vi "Periodic Tasks.vi"(8 "error in":errorcluster) -> ()   [LabVIEW 2013]
doc: "This VI runs in parallel to other tasks. It can contain as many user-defined periodic loops as you need. These can carry out PID or other sorts of timed response."
uses:
  <vilib>/Rock Robotics/WPI/Relay/WPI_RelayValue.ctl
  <vilib>/Rock Robotics/WPI/Solenoid/WPI_SolenoidValue.ctl
  <vilib>/Rock Robotics/WPI/Solenoid/WPI_SolenoidSetEnum.vi
  <vilib>/Rock Robotics/WPI/Solenoid/WPI_SolenoidGet.vi
  <vilib>/Rock Robotics/WPI/Solenoid/WPI_SolenoidGetEnum.vi
  <vilib>/Rock Robotics/WPI/Solenoid/Deprecated/WPI_SolenoidGetBool.vi
  <vilib>/Rock Robotics/WPI/RobotDrive/WPI_RobotDriveGetSetRefNum.vi
  Sample and Hold.vi
  <vilib>/addons/control/pid/pid.llb/PID (DBL).vi
  Stable.vi
  <vilib>/Rock Robotics/WPI/RobotDrive/WPI_RobotDriveMecanumDrive_Cartesian.vi
  <vilib>/Rock Robotics/SystemInterfaces/Utilities/FPGA_UtilitiesLED Source.ctl
  <vilib>/Rock Robotics/SystemInterfaces/Utilities/FPGA_UtilitiesLED State.ctl
  Robot Global Data.vi
  <vilib>/addons/control/pid/NI_PID_pid.lvlib
panel:
  in  "Eval Period (sec)":dbl(knob)=0.1607904282898374 scale=0.0..1.0
  in  "Tab Control 2":T1(tab)
  out "Left 2":dbl(graph)
  out "Perpendicular Distance to Ball 2":dbl(graph)
  out "Right 2":dbl(graph)
  in  "Sonar Offset 2":dbl
  in  "Sonar Scale 2":dbl(knob)=103.01876216940353 scale=0.0..120.0
  in  "Reset Sonar 2":bool
  in  "Kick Sonar 2":bool
  in  "milliseconds to wait":u32=100
  in  "Turn Time 2":dbl
  in  "Turn 2":dbl
  in  "Left Turn Offset 2":dbl
  out "Angle 2":dbl(graph)
  out "Direction 2":bool
  out "Ball Y 2":sgl
  out "Ball X 2":sgl
  in  "Tank Test":bool
  in  "Base":dbl step=0.1
  in  "PID gains":T2={"proportional gain (Kc)"=0.04, "integral time (Ti, min)"=0.010000000000000009, "derivative time (Td, min)"=0.001} {"derivative time (Td, min)" format="%.3f"; "integral time (Ti, min)" format="%.3f"; "proportional gain (Kc)" format="%.3f"}
  in  "Limit":dbl=0.8 format="%#_13g"
  out "Auto Turn Error":dbl
  out "Save Drive":bool
  in  "Burst":i32=75
  in  "loop period (ms) 2":u32=200
  in  "Log Enable":bool
  out "yawGyro 2":dbl(knob) scale=-180.0..180.0
  out "yawGyro":dbl
  in  "Pass Motor Value":dbl
  in  "Load Intake Motor Value":dbl
  out "Stable":bool
  in  "Tab Control":T3(tab)
  out "Left":dbl(graph)
  out "Perpendicular Distance to Ball":dbl(graph)
  out "Right":dbl(graph)
  in  "Sonar Offset":dbl
  in  "Sonar Scale":dbl(knob)=103.01876216940353 scale=0.0..120.0
  in  "Reset Sonar":bool
  in  "Kick Sonar":bool
  in  "Roate PID":T2={"proportional gain (Kc)"=0.04, "integral time (Ti, min)"=0.0, "derivative time (Td, min)"=0.001} {"derivative time (Td, min)" format="%.3f"; "integral time (Ti, min)" format="%.3f"; "proportional gain (Kc)" format="%.3f"}
  in  "Reset Gyro":bool
  in  "Turn Time":dbl
  in  "Turn":dbl
  in  "Left Turn Offset":dbl
  out "Angle":dbl(graph)
  out "Direction":bool
  out "Valid Target":bool
  out "Ball Y":sgl
  out "Ball X":sgl
  out "Valid Ball":bool
  out "Ball X":dbl(graph)
  in  "Track PID":T2={"proportional gain (Kc)"=0.04, "integral time (Ti, min)"=0.0, "derivative time (Td, min)"=0.001} {"derivative time (Td, min)" format="%.3f"; "integral time (Ti, min)" format="%.3f"; "proportional gain (Kc)" format="%.3f"}
  in  "Stop Rotate PID":T2={"proportional gain (Kc)"=0.04, "integral time (Ti, min)"=0.0, "derivative time (Td, min)"=0.001} {"derivative time (Td, min)" format="%.3f"; "integral time (Ti, min)" format="%.3f"; "proportional gain (Kc)" format="%.3f"}
  out "IR Test LED":bool
  # "True is turn\nFalse is drive"
  # "Auto Turn"
  # "Auto Turn"
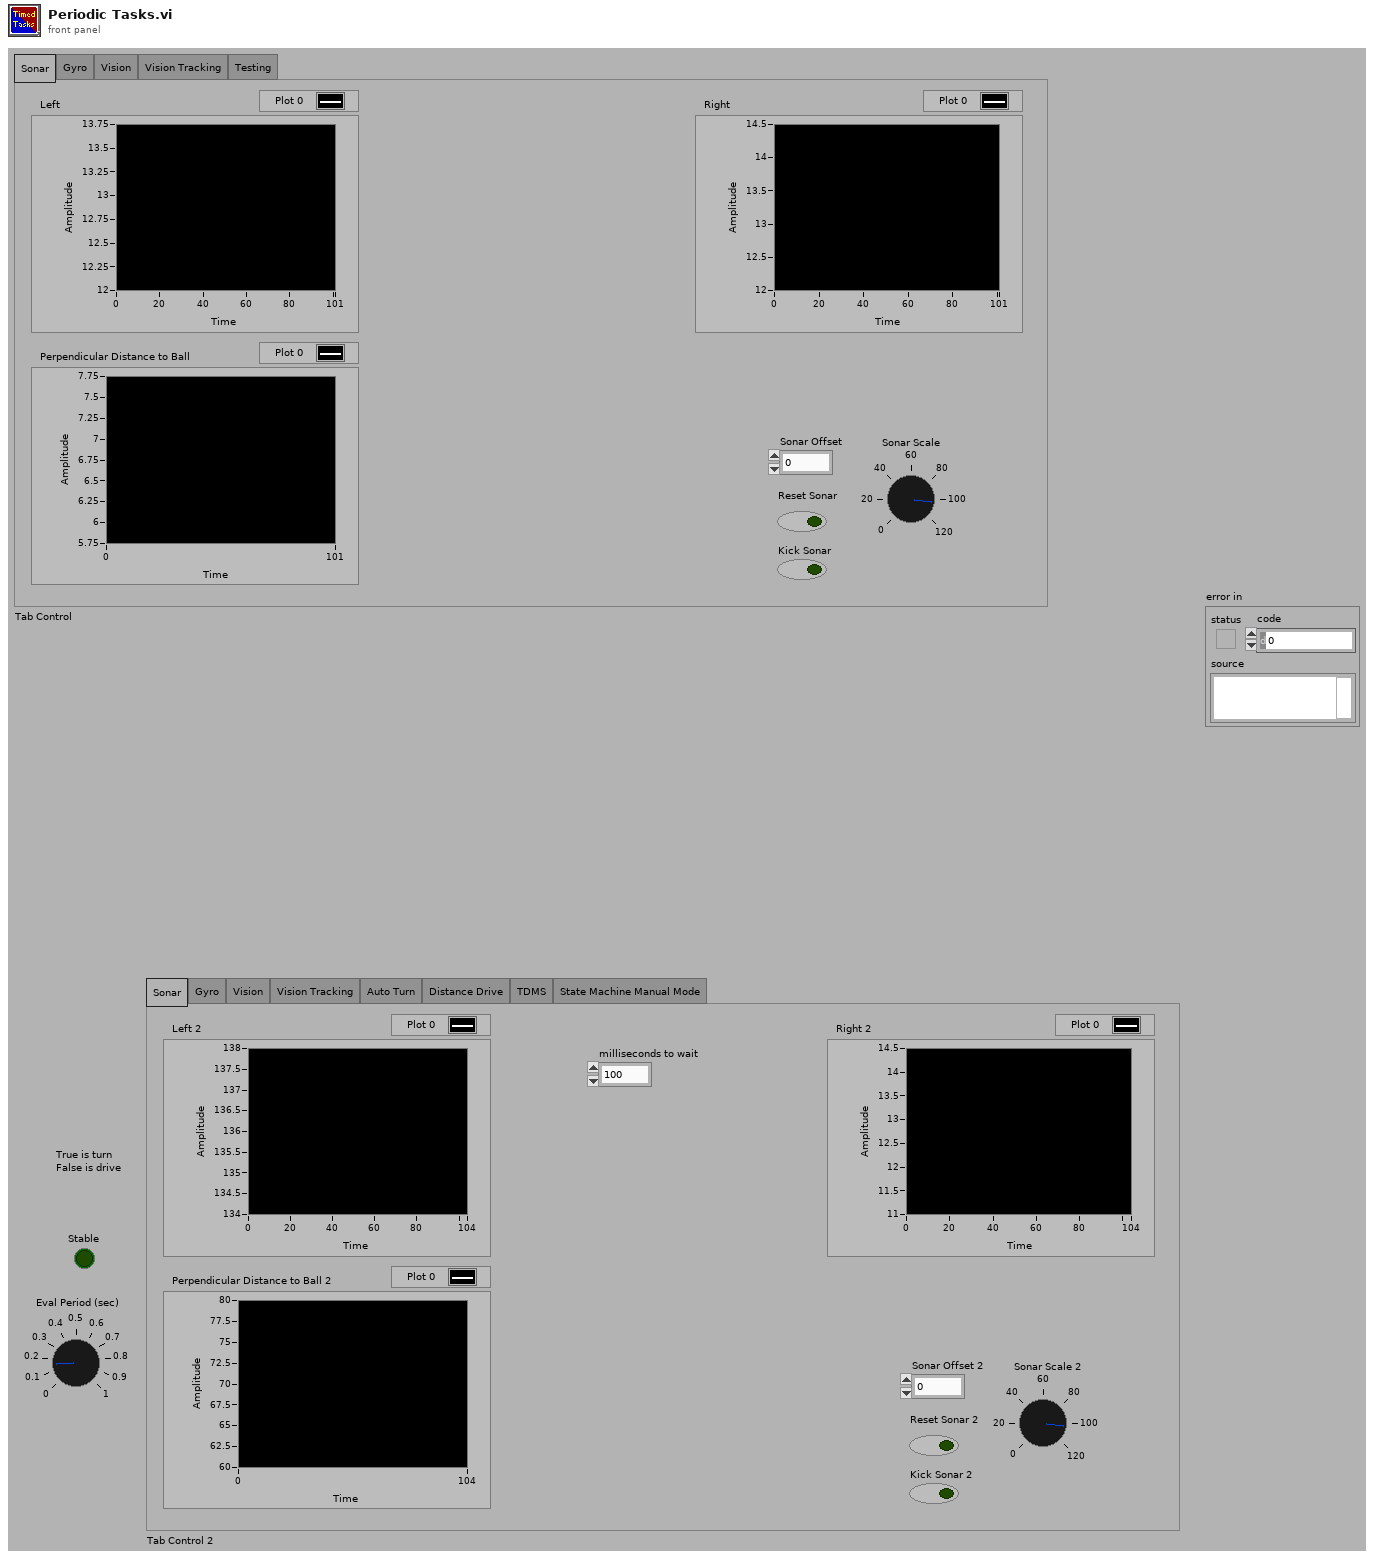
[diagram p1: front panel]
types:
  T1 = enum32{"Sonar", "Gyro", "Vision", "Vision Tracking", "Auto Turn", "Distance Drive", "TDMS", "State Machine Manual Mode"}
  T2 = cluster{"proportional gain (Kc)":dbl, "integral time (Ti, min)":dbl, "derivative time (Td, min)":dbl}
  T3 = enum32{"Sonar", "Gyro", "Vision", "Vision Tracking", "Testing"}
  T4 = enum16{"open", "open or create", "create or replace", "create", "open (read-only)"}
  T5 = typedef "FPGA_UtilitiesLED State.ctl" = enum16{"Off", "On", "Toggle"}
  T6 = typedef "FPGA_UtilitiesLED Source.ctl" = enum16{"User LED", "FPGA LED"}
  T7 = typedef "WPI_JoystickDevRef.ctl" = cluster{"Device":T8}
  T8 = typedef "WPI_JoystickDeviceEnum.ctl" = enum16{"USB 1", "USB 2", "USB 3", "USB 4", "Kinect 1", "Kinect 2"}
  T9 = typedef "WPI_RobotDriveDevRef.ctl" = cluster{"DevStatus":errorcluster, "Motors[]":T10[], "Square Inputs":bool, "Max Output":dbl, "Isochronous":bool}
  T10 = typedef "WPI_MotorControlDeviceRef.ctl" = cluster{"DeviceStatus":errorcluster, "Type":enum16{"PWM", "CAN"}, "PWM":cluster{"Digital Module":T11, "PWM Channel":T12, "DeadBand":T13}, "CAN":cluster{"Device Number":u8, "Control Mode":T14, "Semaphore":T15, "Max Vout":dbl}, "Invert":bool, "TransformRef":T16, "InvTransformRef":T16}
  T11 = typedef "FPGA_TypedefDigitalModule.ctl" = enum16{"Digital Module 1", "Digital Module 2"}
  T12 = typedef "FPGA_DIOPWMChannel.ctl" = enum8{"PWM 1", "PWM 2", "PWM 3", "PWM 4", "PWM 5", "PWM 6", "PWM 7", "PWM 8", "PWM 9", "PWM 10", "Invalid"}
  T13 = typedef "WPI_PWMDeadband.ctl" = cluster{"Name":string, "maxPositivePwm":i32, "minPositivePwm":i32, "centerPwm":i32, "maxNegativePwm":i32, "minNegativePwm":i32, "angularRange":u16}
  T14 = typedef "WPI_CANJaguar_ControlMode.ctl" = enum8{"Percent VBus", "Current", "Speed", "Position", "Voltage"}
  T15 = typedef "Semaphore RefNum" = refnum<k1>
  T16 = typedef "WPI_PWMTransform_ConPane.ctl" = refnum<vi>
  T17 = cluster{"JoystickDevRef":T7, "RobotDriveDevRef":T9}
  T18 = typedef "WPI_RelayValue.ctl" = enum16{"Off", "On", "Forward", "Reverse"}
  T19 = typedef "WPI_RelayDevRef.ctl" = cluster{"DevStatus":errorcluster, "Relay Channel":T20, "Digital Module":T11, "Relay Direction":T21}
  T20 = typedef "FPGA_DIORelayChannel.ctl" = enum8{"Relay 1", "Relay 2", "Relay 3", "Relay 4", "Relay 5", "Relay 6", "Relay 7", "Relay 8", "Invalid"}
  T21 = typedef "WPI_RelayDirection.ctl" = enum16{"Both directions", "Forward only", "Reverse only"}
  T22 = typedef "WPI_AnalogChannelDevRef.ctl" = cluster{"DevStatus":errorcluster, "Analog Module":T23, "Analog Channel":T24}
  T23 = typedef "FPGA_TypedefAnalogModule.ctl" = enum16{"Analog Module 1", "Analog Module 2"}
  T24 = typedef "FPGA_AIChannel.ctl" = enum8{"AI 1", "AI 2", "AI 3", "AI 4", "AI 5", "AI 6", "AI 7", "AI 8", "Invalid"}
  T25 = typedef "WPI_DigitalInputDevRef.ctl" = cluster{"DevStatus":errorcluster, "DIO Channel":T26, "Digital Module":T11}
  T26 = typedef "FPGA_DIOChannel.ctl" = enum8{"DIO 1", "DIO 2", "DIO 3", "DIO 4", "DIO 5", "DIO 6", "DIO 7", "DIO 8", "DIO 9", "DIO 10", "DIO 11", "DIO 12", "DIO 13", "DIO 14", "Invalid"}
  T27 = typedef "WPI_SolenoidDevRef.ctl" = cluster{"DevStatus":errorcluster, "Solenoid Module":T28, "Forward Solenoid Channel":T29, "Reverse Solenoid Channel":T29}
  T28 = typedef "FPGA_TypedefSolenoidModule.ctl" = enum16{"Solenoid Module 1", "Solenoid Module 2"}
  T29 = typedef "WPI_SolenoidChannel.ctl" = enum8{"Solenoid 1", "Solenoid 2", "Solenoid 3", "Solenoid 4", "Solenoid 5", "Solenoid 6", "Solenoid 7", "Solenoid 8", "Invalid"}
  T30 = typedef "WPI_SolenoidValue.ctl" = enum16{"Off", "On", "Forward", "Reverse"}
  T31 = typedef "WPI_GyroDevRef.ctl" = cluster{"DevStatus":errorcluster, "Analog Module":T23, "Analog Channel":T24, "Offset":dbl, "Gain (VoltsPerDegree/Second)":dbl}
  T32 = enum16{"Drive", "Rotate", "Track X", "Distance Drive"}
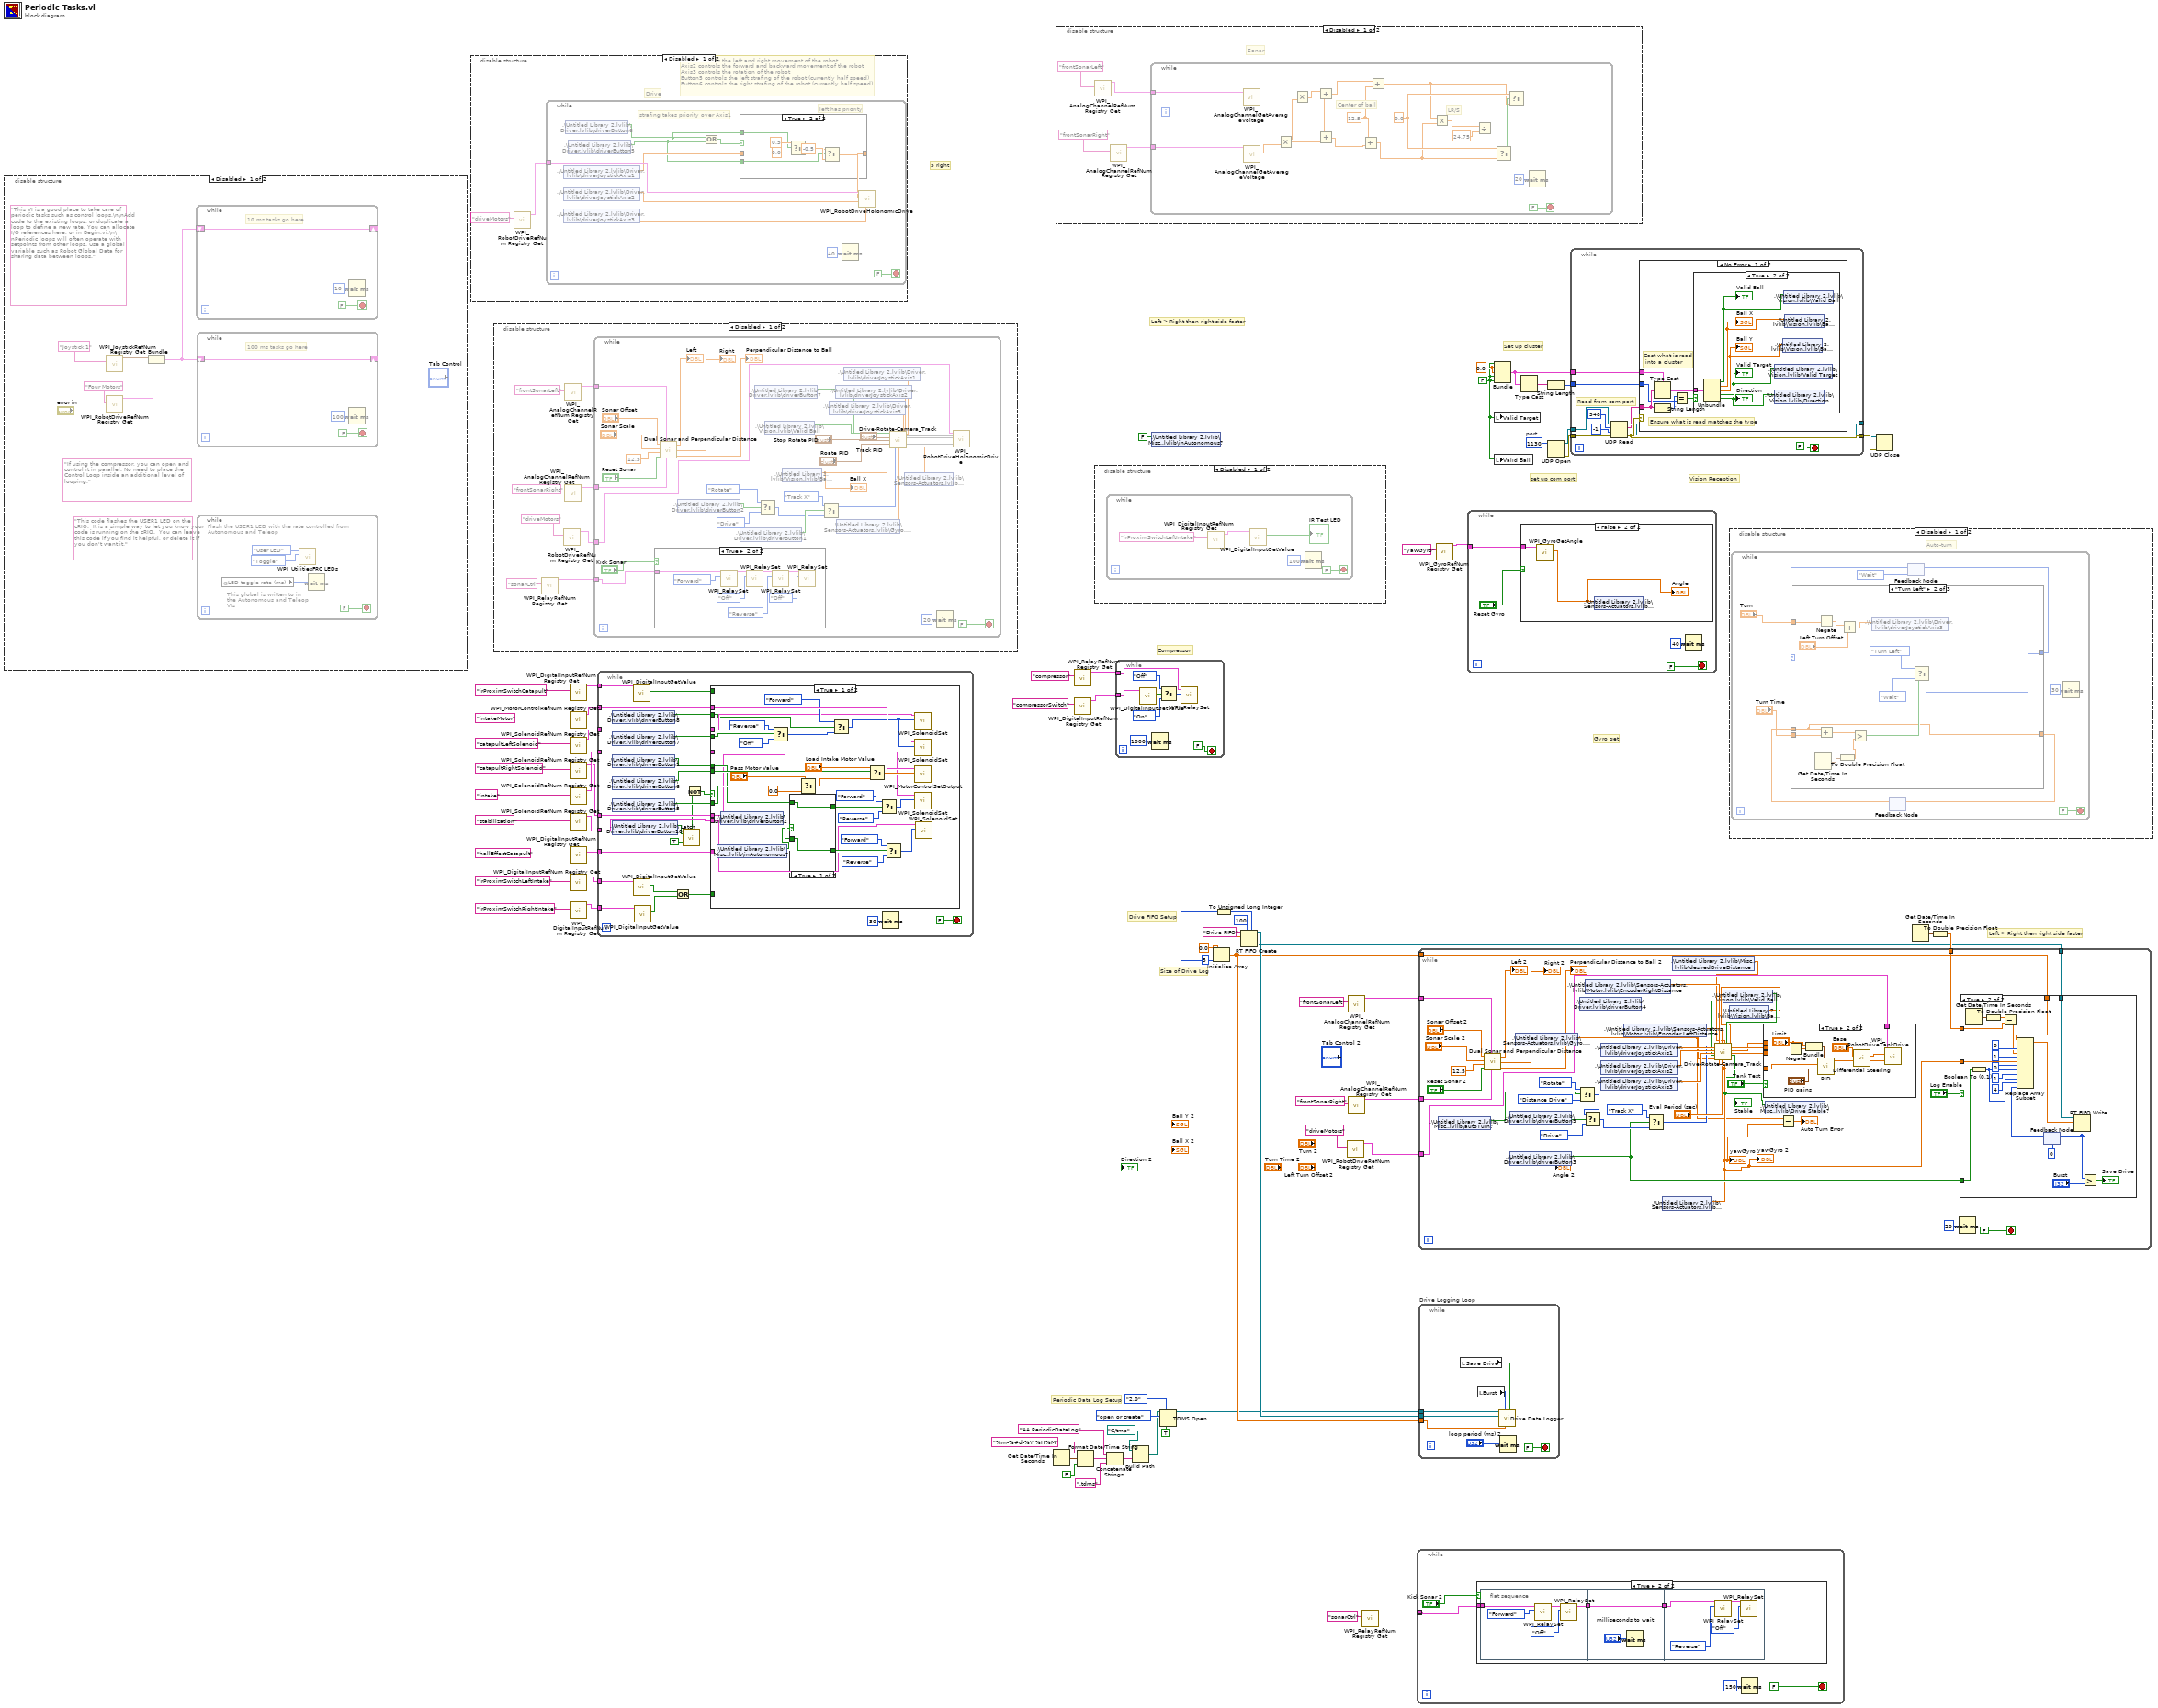
[diagram p0: block diagram]
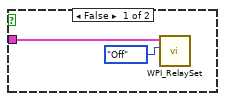
[diagram p2: hidden frame]
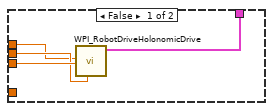
[diagram p4: hidden frame]
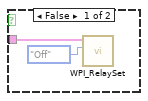
[diagram p5: hidden frame]
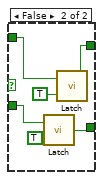
[diagram p7: hidden frame]
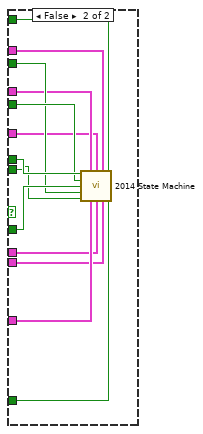
[diagram p8: hidden frame]
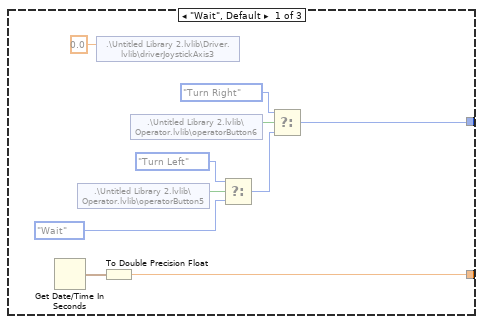
[diagram p10: hidden frame]
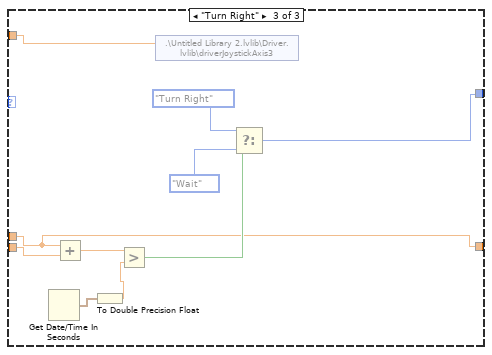
[diagram p11: hidden frame]
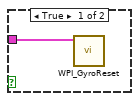
[diagram p13: hidden frame]
diagram:
  w31 = 5 ("dimension size")
  w58 = sgl 0.0
  w56 = FALSE
  w65 = u16 1130  # port
  # "Periodic Data Log Setup"
  # "Drive FIFO Setup"
  # "Size of Drive Log"
  # "Left > Right then right side faster"
  # "Compressor"
  # "Vision Reception"
  # "Gyro get"
  # "Left > Right then right side faster"
  # "set up com port"
  # "Set up cluster"
  # "5 right"
  n1 = disable-structure shown="Disabled" {
    frame Disabled {
      (unwired) "If using the compressor, you can open and control it in parallel. No need to place the Control Loop inside an additional level of looping."
      (unwired) "This code flashes the USER1 LED on the cRIO.  It is a simple way to let you know your code is running on the cRIO.  You can leave this code if you find it helpful, or delete it if you don't want it."
      (unwired) "This VI is a good place to take care of periodic tasks such as control loops.\n\nAdd code to the existing loops, or duplicate a loop to define a new rate. You can allocate I/O references here, or in Begin.vi.\n\nPeriodic loops will often operate with setpoints from other loops. Use a global variable such as Robot Global Data for sharing data between loops."
      n2 = call <vilib>:"WPI_JoystickRefNum Registry Get.vi"("refnum name"="Joystick 1") -> ("JoystickDevRef"=w68:T7)  [unwired: 1 in, 9 out]
      n3 = call <vilib>:"WPI_RobotDriveRefNum Registry Get.vi"("refnum name"="Four Motors") -> ("RobotDriveDevRef"=w67:T9)  [unwired: 1 in, 9 out]
      n4 = Bundle("JoystickDevRef"=w68, "RobotDriveDevRef"=w67) -> (w66:T17)  [unwired: 1 out]
      n5 = while {
        shift-right: [w78] -> _
        shift-left: w66 -> [w78]
        stop <- FALSE stop-if-true
        # "10 ms tasks go here"
        n6 = Wait (ms)(milliseconds to wait=u32 10) -> ()  [unwired: 1 out]
      }
      n7 = while {
        shift-right: [w75] -> _
        shift-left: w66 -> [w75]
        stop <- FALSE stop-if-true
        # "100 ms tasks go here"
        n8 = Wait (ms)(milliseconds to wait=u32 100) -> ()  [unwired: 1 out]
      }
      n9 = while {
        stop <- FALSE stop-if-true
        # "This global is written to in the Autonomous and Teleop VIs"
        # "Flash the USER1 LED with the rate controlled from Autonomous and Teleop"
        n10 = global read "Robot Global Data.vi" "LED toggle rate (ms)"() -> (w71:u32)
        n11 = call <vilib>:"WPI_UtilitiesFRC LEDs.vi"("State"=FPGA_UtilitiesLED_State."Toggle", "LED Type"=FPGA_UtilitiesLED_Source."User LED") -> ()  [unwired: 1 in, 9 out]
        n12 = Wait (ms)(milliseconds to wait=w71) -> ()  [unwired: 1 out]
      }
    }
    frame Enabled {
    }
  }
  n13 = disable-structure shown="Disabled" {
    frame Disabled {
      # "Axis1 controls the left and right movement of the robot\nAxis2 controls the forward and backward movement of the robot\nAxis3 controls the rotation of the robot\nButton5 controls the left strafing of the robot (currently half speed)\nButton6 controls the right strafing of the robot (currently half speed)"
      # "Drive"
      n14 = call <vilib>:"WPI_RobotDriveRefNum Registry Get.vi"("refnum name"="driveMotors") -> ("RobotDriveDevRef"=w82:T9)  [unwired: 9 in, 1 out]
      n15 = while {
        tunnel: w82 -> [w91]
        stop <- FALSE stop-if-true
        # "left has priority"
        # "strafing takes priority over Axis1"
        n16 = shared-variable ".\\Untitled Library 2.lvlib\\Driver.lvlib\\driverJoystickAxis1"() -> (w86:dbl)  [unwired: 1 in, 1 out]
        n17 = shared-variable ".\\Untitled Library 2.lvlib\\Driver.lvlib\\driverJoystickAxis2"() -> (w90:dbl)  [unwired: 1 in, 1 out]
        n18 = shared-variable ".\\Untitled Library 2.lvlib\\Driver.lvlib\\driverJoystickAxis3"() -> (w89:dbl)  [unwired: 1 in, 1 out]
        n19 = shared-variable ".\\Untitled Library 2.lvlib\\Driver.lvlib\\driverButton6"() -> (w85:bool)  [unwired: 1 in, 1 out]
        n20 = shared-variable ".\\Untitled Library 2.lvlib\\Driver.lvlib\\driverButton5"() -> (w84:bool)  [unwired: 1 in, 1 out]
        n21 = Or(x=w85, y=w84) -> (x .or. y?=w88:bool)
        n22 = case shown="True" w88 {
          tunnel: [w93 w96] -> w87
          tunnel: w86 -> [w93 _]
          tunnel: w85 -> [_ w95]
          tunnel: w84 -> [_ w94]
          frame False {
          }
          frame True {
            n23 = Select(t=0.5, s=w95, f=0.0) -> (s? t:f=w98:dbl)
            n24 = Select(t=-0.5, s=w94, f=w98) -> (s? t:f=w96:dbl)
          }
        }
        n25 = Wait (ms)(milliseconds to wait=u32 40) -> ()  [unwired: 1 out]
        n26 = call-poly <vilib>:"WPI_RobotDriveHolonomicDrive.vi"("Rotation"=w89, "Y"=w90, "X"=w87, "RobotDriveDevRef"=w91) -> ()  [unwired: 5 in, 3 out]
      }
    }
    frame Enabled {
    }
  }
  n27 = disable-structure shown="Disabled" {
    frame Disabled {
      n28 = call <vilib>:"WPI_RelayRefNum Registry Get.vi"("refnum name"="sonarCtrl") -> ("RelayDevRef"=w101:T19)  [unwired: 9 in, 1 out]
      n29 = call <vilib>:"WPI_RobotDriveRefNum Registry Get.vi"("refnum name"="driveMotors") -> ("RobotDriveDevRef"=w107:T9)  [unwired: 9 in, 1 out]
      n30 = call <vilib>:"WPI_AnalogChannelRefNum Registry Get.vi"("refnum name"="frontSonarLeft") -> ("AIDeviceRef"=w104:T22)  [unwired: 9 in, 1 out]
      n31 = call <vilib>:"WPI_AnalogChannelRefNum Registry Get.vi"("refnum name"="frontSonarRight") -> ("AIDeviceRef"=w103:T22)  [unwired: 9 in, 1 out]
      n32 = while {
        tunnel: w107 -> [w130]
        tunnel: w104 -> [w143]
        tunnel: w103 -> [w142]
        tunnel: w101 -> [w132]
        stop <- FALSE stop-if-true
        n33 = case shown="True" "Kick Sonar" {
          tunnel: w132 -> [w145 w149]
          frame False {
            n34 = call <vilib>:"WPI_RelaySet.vi"("RelayValue"=WPI_RelayValue."Off", "RelayDevRef"=w145) -> ()  [unwired: 8 in, 2 out]
          }
          frame True {
            n35 = call <vilib>:"WPI_RelaySet.vi"("RelayValue"=WPI_RelayValue."Forward", "RelayDevRef"=w149) -> ("RelayDevRef"=w147:T19)  [unwired: 8 in, 1 out]
            n36 = call <vilib>:"WPI_RelaySet.vi"("RelayValue"=WPI_RelayValue."Off", "RelayDevRef"=w147) -> ("RelayDevRef"=w148:T19)  [unwired: 8 in, 1 out]
            n37 = call <vilib>:"WPI_RelaySet.vi"("RelayValue"=WPI_RelayValue."Reverse", "RelayDevRef"=w148) -> ("RelayDevRef"=w150:T19)  [unwired: 8 in, 1 out]
            n38 = call <vilib>:"WPI_RelaySet.vi"("RelayValue"=WPI_RelayValue."Off", "RelayDevRef"=w150) -> ()  [unwired: 8 in, 2 out]
          }
        }
        n39 = call "Dual Sonar and Perpendicular Distance.vi"("Sonar Offset"="Sonar Offset", "Left Sonar Dev Ref"=w143, "Sonar Scale"="Sonar Scale", "Radius of Ball"=12.5, "Right Sonar Dev Ref"=w142, "ResetSonar"="Reset Sonar") -> ("Left"=→"Left":dbl, "Right"=→"Right":dbl, "Perpendicular Distance to Ball"=→"Perpendicular Distance to Ball":dbl)
        n40 = shared-variable ".\\Untitled Library 2.lvlib\\Driver.lvlib\\driverButton2"() -> (w118:bool)  [unwired: 1 in, 1 out]
        n41 = shared-variable ".\\Untitled Library 2.lvlib\\Driver.lvlib\\driverButton1"() -> (w117:bool)  [unwired: 1 in, 1 out]
        n42 = shared-variable ".\\Untitled Library 2.lvlib\\Driver.lvlib\\driverButton7"() -> (w119:bool)  [unwired: 1 in, 1 out]
        n43 = Select(t=enum16{"Drive", "Rotate", "Track X"}."Rotate" ("State"), s=w118, f=enum16{"Drive", "Rotate", "Track X"}."Drive" ("State")) -> (s? t:f=w113:enum16{"Drive", "Rotate", "Track X"})
        n44 = shared-variable ".\\Untitled Library 2.lvlib\\Vision.lvlib\\Valid Ball"() -> (w120:bool)  [unwired: 1 in, 1 out]
        n45 = shared-variable ".\\Untitled Library 2.lvlib\\Vision.lvlib\\Ball X"() -> (w110:dbl)  [unwired: 1 in, 1 out]
        "Ball X" <- w110
        n46 = Select(t=enum16{"Drive", "Rotate", "Track X"}."Track X" ("State"), s=w117, f=w113) -> (s? t:f=w114:enum16{"Drive", "Rotate", "Track X"})
        n47 = shared-variable ".\\Untitled Library 2.lvlib\\Driver.lvlib\\driverJoystickAxis3"() -> (w124:dbl)  [unwired: 1 in, 1 out]
        n48 = shared-variable ".\\Untitled Library 2.lvlib\\Driver.lvlib\\driverJoystickAxis2"() -> (w125:dbl)  [unwired: 1 in, 1 out]
        n49 = shared-variable ".\\Untitled Library 2.lvlib\\Sensors-Actuators.lvlib\\Gyro.lvlib\\Desired Angle"() -> (w109:dbl)  [unwired: 1 in, 1 out]
        n50 = shared-variable ".\\Untitled Library 2.lvlib\\Driver.lvlib\\driverJoystickAxis1"() -> (w126:dbl)  [unwired: 1 in, 1 out]
        n51 = shared-variable ".\\Untitled Library 2.lvlib\\Sensors-Actuators.lvlib\\Gyro.lvlib\\yawGyro"() -> (w111:dbl)  [unwired: 1 in, 1 out]
        n52 = call "Drive-Rotate-Camera_Track.vi"(0:w124, 5:w125, 6:w109, 7:w126, 8:w111, 9:w119, 10:w114, 11:w120, 12:"Track PID", 13:"Stop Rotate PID", 14:"Roate PID", 15:w110) -> (1:w129, 2:w128, 3:w127)  [unwired: 1 in]
        n53 = Wait (ms)(milliseconds to wait=u32 20) -> ()  [unwired: 1 out]
        n54 = call-poly <vilib>:"WPI_RobotDriveHolonomicDrive.vi"("Rotation"=w127, "Y"=w128, "X"=w129, "RobotDriveDevRef"=w130) -> ()  [unwired: 5 in, 3 out]
      }
    }
    frame Enabled {
    }
  }
  n55 = call <vilib>:"WPI_DigitalInputRefNum Registry Get.vi"("refnum name"="irProximSwitchCatapult") -> ("DigitalInputDevRef"=w44:T25)  [unwired: 9 in, 1 out]
  n56 = call <vilib>:"WPI_MotorControlRefNum Registry Get.vi"("refnum name"="intakeMotor") -> ("MotorControlDevRef"=w6:T10)  [unwired: 9 in, 1 out]
  n57 = call <vilib>:"WPI_SolenoidRefNum Registry Get.vi"("refnum name"="catapultLeftSolenoid") -> ("SolenoidDevRef"=w5:T27)  [unwired: 9 in, 1 out]
  n58 = call <vilib>:"WPI_SolenoidRefNum Registry Get.vi"("refnum name"="catapultRightSolenoid") -> ("SolenoidDevRef"=w2:T27)  [unwired: 9 in, 1 out]
  n59 = call <vilib>:"WPI_SolenoidRefNum Registry Get.vi"("refnum name"="intake") -> ("SolenoidDevRef"=w3:T27)  [unwired: 9 in, 1 out]
  n60 = call <vilib>:"WPI_SolenoidRefNum Registry Get.vi"("refnum name"="stabilization") -> ("SolenoidDevRef"=w4:T27)  [unwired: 9 in, 1 out]
  n61 = call <vilib>:"WPI_DigitalInputRefNum Registry Get.vi"("refnum name"="hallEffectCatapult") -> ("DigitalInputDevRef"=w42:T25)  [unwired: 9 in, 1 out]
  n62 = call <vilib>:"WPI_DigitalInputRefNum Registry Get.vi"("refnum name"="irProximSwitchLeftIntake") -> ("DigitalInputDevRef"=w46:T25)  [unwired: 9 in, 1 out]
  n63 = call <vilib>:"WPI_DigitalInputRefNum Registry Get.vi"("refnum name"="irProximSwitchRightIntake") -> ("DigitalInputDevRef"=w45:T25)  [unwired: 9 in, 1 out]
  n64 = while {
    tunnel: w46 -> [w176]
    tunnel: w45 -> [w175]
    tunnel: w44 -> [w174]
    tunnel: w42 -> [w162]
    tunnel: w6 -> [w161]
    tunnel: w5 -> [w160]
    tunnel: w2 -> [w159]
    tunnel: w4 -> [w158]
    tunnel: w3 -> [w157]
    stop <- FALSE stop-if-true
    n65 = shared-variable ".\\Untitled Library 2.lvlib\\Driver.lvlib\\driverButton8"() -> (w169:bool)  [unwired: 1 in, 1 out]
    n66 = shared-variable ".\\Untitled Library 2.lvlib\\Driver.lvlib\\driverButton7"() -> (w168:bool)  [unwired: 1 in, 1 out]
    n67 = shared-variable ".\\Untitled Library 2.lvlib\\Driver.lvlib\\driverButton1"() -> (w165:bool)  [unwired: 1 in, 1 out]
    n68 = shared-variable ".\\Untitled Library 2.lvlib\\Driver.lvlib\\driverButton6"() -> (w167:bool)  [unwired: 1 in, 1 out]
    n69 = shared-variable ".\\Untitled Library 2.lvlib\\Driver.lvlib\\driverButton5"() -> (w166:bool)  [unwired: 1 in, 1 out]
    n70 = shared-variable ".\\Untitled Library 2.lvlib\\Driver.lvlib\\driverButton10"() -> (w164:bool)  [unwired: 1 in, 1 out]
    n71 = call <vilib>:"WPI_DigitalInputGetValue.vi"("DigitalInputDevRef"=w174) -> ("Value"=w170:bool)  [unwired: 8 in, 2 out]
    n72 = call <vilib>:"WPI_DigitalInputGetValue.vi"("DigitalInputDevRef"=w176) -> ("Value"=w173:bool)  [unwired: 8 in, 2 out]
    n73 = call <vilib>:"WPI_DigitalInputGetValue.vi"("DigitalInputDevRef"=w175) -> ("Value"=w172:bool)  [unwired: 8 in, 2 out]
    n74 = Or(x=w173, y=w172) -> (x .or. y?=w171:bool)
    n75 = call "Latch.vi"("Edge"=TRUE, "In"=w164) -> ("Out"=w154:bool)
    n76 = Not(x=w154) -> (.not. x?=w155:bool)
    n77 = case shown="True" w155 {
      tunnel: w171 -> [_ w222]
      tunnel: w170 -> [_ w223]
      tunnel: w169 -> [w180 w225]
      tunnel: w168 -> [w198 w227]
      tunnel: w167 -> [w207 w224]
      tunnel: w166 -> [w206 w226]
      tunnel: w165 -> [w188 w228]
      tunnel: w162 -> [_ w221]
      tunnel: w161 -> [w203 w220]
      tunnel: w160 -> [w194 w219]
      tunnel: w159 -> [w182 w218]
      tunnel: w158 -> [w179 w217]
      tunnel: w157 -> [w181 w216]
      frame True {
        n78 = shared-variable ".\\Untitled Library 2.lvlib\\Misc..lvlib\\inAutonomous?"() -> (w178:bool)  [unwired: 1 in, 1 out]
        n79 = shared-variable ".\\Untitled Library 2.lvlib\\Driver.lvlib\\driverButton2"() -> (w185:bool)  [unwired: 1 in, 1 out]
        n80 = Select(t=WPI_SolenoidValue."Reverse" ("Value"), s=w198, f=WPI_SolenoidValue."Off" ("Value")) -> (s? t:f=w199:T30)
        n81 = case shown="True" w178 {
          tunnel: [w209 w214] -> w190
          tunnel: w188 -> [w209 w213]
          tunnel: [w208 w211] -> w186
          tunnel: w185 -> [w208 w210]
          frame True {
          }
          frame False {
            n82 = call "Latch.vi"("Edge"=TRUE, "In"=w210) -> ("Out"=w211:bool)
            n83 = call "Latch.vi"("Edge"=TRUE, "In"=w213) -> ("Out"=w214:bool)
          }
        }
        n84 = Select(t="Pass Motor Value", s=w206, f=0.0) -> (s? t:f=w205:dbl)
        n85 = Select(t=WPI_SolenoidValue."Forward" ("Value"), s=w180, f=w199) -> (s? t:f=w193:T30)
        n86 = Select(t="Load Intake Motor Value", s=w207, f=w205) -> (s? t:f=w204:dbl)
        n87 = Select(t=WPI_SolenoidValue."Forward" ("Value"), s=w190, f=WPI_SolenoidValue."Reverse" ("Value")) -> (s? t:f=w189:T30)
        n88 = Select(t=WPI_SolenoidValue."Forward" ("Value"), s=w186, f=WPI_SolenoidValue."Reverse" ("Value")) -> (s? t:f=w183:T30)
        n89 = call-poly <vilib>:"WPI_SolenoidSet.vi"("Value"=w193, "SolenoidDevRef"=w194) -> ()  [unwired: 8 in, 2 out]
        n90 = call-poly <vilib>:"WPI_SolenoidSet.vi"("Value"=w193, "SolenoidDevRef"=w182) -> ()  [unwired: 8 in, 2 out]
        n91 = call <vilib>:"WPI_MotorControlSetOutput.vi"("Output"=w204, "MotorControlDevRef"=w203) -> ()  [unwired: 7 in, 3 out]
        n92 = call-poly <vilib>:"WPI_SolenoidSet.vi"("Value"=w189, "SolenoidDevRef"=w181) -> ()  [unwired: 8 in, 2 out]
        n93 = call-poly <vilib>:"WPI_SolenoidSet.vi"("Value"=w183, "SolenoidDevRef"=w179) -> ()  [unwired: 8 in, 2 out]
      }
      frame False {
        n94 = call "2014 State Machine.vi"("Toggle Robot Open/Close"=w228, "Left Catapult Solenoid Refnum"=w219, "Intake Solenoid Refnum"=w216, "Intake Motor Refnum"=w220, "Ball in launcher"=w223, "Shoot Over Truss"=w227, "Pass"=w226, "Shoot for the Goal"=w225, "Intake Load"=w224, "Hall Effect Catapult"=w221, "Right Catapult Solenoid Refnum"=w218, "Stabilizer Refnum"=w217, "Ball in intake"=w222) -> ()  [unwired: 3 in]
      }
    }
    n95 = Wait (ms)(milliseconds to wait=u32 30) -> ()  [unwired: 1 out]
  }
  n96 = Get Date/Time In Seconds() -> (seconds since 1Jan1904=w18:timestamp)
  n97 = disable-structure shown="Disabled" {
    frame Disabled {
      # "Sonar"
      n98 = call <vilib>:"WPI_AnalogChannelRefNum Registry Get.vi"("refnum name"="frontSonarLeft") -> ("AIDeviceRef"=w232:T22)  [unwired: 9 in, 1 out]
      n99 = call <vilib>:"WPI_AnalogChannelRefNum Registry Get.vi"("refnum name"="frontSonarRight") -> ("AIDeviceRef"=w231:T22)  [unwired: 9 in, 1 out]
      n100 = while {
        tunnel: w232 -> [w253]
        tunnel: w231 -> [w252]
        stop <- FALSE stop-if-true
        w239 = 12.5
        w248 = 0.0
        # "LR/S"
        # "Center of ball"
        n101 = call <vilib>:"WPI_AnalogChannelGetAverageVoltage.vi"("AIDeviceRef"=w253) -> ("Voltage"=w247:dbl)  [unwired: 8 in, 2 out]
        n102 = call <vilib>:"WPI_AnalogChannelGetAverageVoltage.vi"("AIDeviceRef"=w252) -> ("Voltage"=w245:dbl)  [unwired: 8 in, 2 out]
        n103 = Multiply(x=w247) -> (y=w244:dbl, x*y=w246:dbl)
        n104 = Multiply(x=w244, y=w245) -> (x*y=w242:dbl)
        n105 = Add(x=w246) -> (y=w243:dbl, x+y=w241:dbl)
        n106 = Add(x=w243, y=w242) -> (x+y=w240:dbl)
        n107 = Add(x=w239, y=w240) -> (x+y=w236:dbl)
        n108 = Add(x=w241, y=w239) -> (x+y=w237:dbl)
        n109 = Multiply(x=w237, y=w236) -> (x*y=w235:dbl)
        n110 = Divide(x=w235, y=24.75) -> (x/y=w233:dbl)
        n111 = Select(t=w248, f=w236) -> (s=w238:bool, s? t:f=w249:dbl)
        n112 = Select(t=w248, s=w238, f=w237) -> ()  [unwired: 1 out]
        n113 = Wait (ms)(milliseconds to wait=u32 20) -> ()  [unwired: 1 out]
      }
    }
    frame Enabled {
    }
  }
  n114 = call <vilib>:"WPI_RelayRefNum Registry Get.vi"("refnum name"="compressor") -> ("RelayDevRef"=w52:T19)  [unwired: 9 in, 1 out]
  n115 = call <vilib>:"WPI_DigitalInputRefNum Registry Get.vi"("refnum name"="compressorSwitch") -> ("DigitalInputDevRef"=w53:T25)  [unwired: 9 in, 1 out]
  n116 = Format Date/Time String(time format string (%c)="%m-%#d-%Y %H%M", seconds (now)=w18, UTC format=FALSE) -> (date/time string=w23:string)
  n117 = disable-structure shown="Disabled" {
    frame Disabled {
      n118 = while {
        stop <- FALSE stop-if-true
        n119 = call <vilib>:"WPI_DigitalInputRefNum Registry Get.vi"("refnum name"="irProximSwitchLeftIntake") -> ("DigitalInputDevRef"=w257:T25)  [unwired: 9 in, 1 out]
        n120 = call <vilib>:"WPI_DigitalInputGetValue.vi"("DigitalInputDevRef"=w257) -> ("Value"=→"IR Test LED":bool)  [unwired: 8 in, 2 out]
        n121 = Wait (ms)(milliseconds to wait=u32 100) -> ()  [unwired: 1 out]
      }
    }
    frame Enabled {
    }
  }
  n122 = Concatenate Strings("AA PeriodicDataLog" ("string"), w23, ".tdms" ("string")) -> (w24:string)
  n123 = while {
    tunnel: w53 -> [w266]
    tunnel: w52 -> [w265]
    stop <- FALSE stop-if-true
    n124 = call <vilib>:"WPI_DigitalInputGetValue.vi"("DigitalInputDevRef"=w266) -> ("Value"=w264:bool)  [unwired: 8 in, 2 out]
    n125 = Wait (ms)(milliseconds to wait=u32 1000) -> ()  [unwired: 1 out]
    n126 = Select(t=WPI_RelayValue."Off" ("RelayValue"), s=w264, f=WPI_RelayValue."On" ("RelayValue")) -> (s? t:f=w261:T18)
    n127 = call <vilib>:"WPI_RelaySet.vi"("RelayValue"=w261, "RelayDevRef"=w265) -> ()  [unwired: 8 in, 2 out]
  }
  n128 = Build Path(base path=path "C:/tmp" ("file path (dialog if empty)"), name or relative path=w24) -> (appended path=w15:path)
  n129 = shared-variable ".\\Untitled Library 2.lvlib\\Misc..lvlib\\inAutonomous?"(FALSE ("inAutonomous?")) -> ()  [unwired: 1 in, 1 out]
  n130 = TDMS Open(6:TRUE ("disable buffering? (T)"), 7:enum16{"1.0", "2.0"}."2.0" ("file format version (2.0)"), 10:T4."open or create" ("operation (0:open)"), 11:w15) -> (3:w13:refnum<k34>)  [unwired: 3 in, 1 out]
  n131 = Initialize Array(0.0, w31) -> (w25:dbl[])
  n132 = To Unsigned Long Integer(number=w31) -> (unsigned 32bit integer=w30:u32)
  n133 = RT FIFO Create(0:"Drive FIFO" ("name (unnamed)"), 1:w25, 4:u32 100 ("size (10)"), 6:w30) -> (8:w26:refnum<k33>)  [unwired: 4 in, 2 out]
  n134 = call <vilib>:"WPI_RobotDriveRefNum Registry Get.vi"("refnum name"="driveMotors") -> ("RobotDriveDevRef"=w40:T9)  [unwired: 9 in, 1 out]
  n135 = call <vilib>:"WPI_AnalogChannelRefNum Registry Get.vi"("refnum name"="frontSonarLeft") -> ("AIDeviceRef"=w37:T22)  [unwired: 9 in, 1 out]
  n136 = call <vilib>:"WPI_AnalogChannelRefNum Registry Get.vi"("refnum name"="frontSonarRight") -> ("AIDeviceRef"=w36:T22)  [unwired: 9 in, 1 out]
  n137 = call <vilib>:"WPI_RelayRefNum Registry Get.vi"("refnum name"="sonarCtrl") -> ("RelayDevRef"=w34:T19)  [unwired: 9 in, 1 out]
  n138 = while {
    tunnel: [w268] -> _
    tunnel: w34 -> [w268]
    stop <- FALSE stop-if-true
    n139 = case shown="True" "Kick Sonar 2" {
      tunnel: w268 -> [w271 w275]
      frame False {
        n140 = call <vilib>:"WPI_RelaySet.vi"("RelayValue"=WPI_RelayValue."Off", "RelayDevRef"=w271) -> ()  [unwired: 8 in, 2 out]
      }
      frame True {
        n141 = flat-sequence {
          tunnel: w275 -> [w277]
          tunnel: [w276] -> w274
          tunnel: w274 -> [w282]
          tunnel: [w282] -> w273
          tunnel: w273 -> [w283]
          frame #0 {
            n142 = call <vilib>:"WPI_RelaySet.vi"("RelayValue"=WPI_RelayValue."Forward", "RelayDevRef"=w277) -> ("RelayDevRef"=w279:T19)  [unwired: 8 in, 1 out]
            n143 = call <vilib>:"WPI_RelaySet.vi"("RelayValue"=WPI_RelayValue."Off", "RelayDevRef"=w279) -> ("RelayDevRef"=w276:T19)  [unwired: 8 in, 1 out]
          }
          frame #1 {
            n144 = Wait (ms)(milliseconds to wait="milliseconds to wait") -> ()  [unwired: 1 out]
          }
          frame #2 {
            n145 = call <vilib>:"WPI_RelaySet.vi"("RelayValue"=WPI_RelayValue."Reverse", "RelayDevRef"=w283) -> ("RelayDevRef"=w284:T19)  [unwired: 8 in, 1 out]
            n146 = call <vilib>:"WPI_RelaySet.vi"("RelayValue"=WPI_RelayValue."Off", "RelayDevRef"=w284) -> ()  [unwired: 8 in, 2 out]
          }
        }
      }
    }
    n147 = Wait (ms)(milliseconds to wait=u32 150) -> ()  [unwired: 1 out]
  }
  n148 = while "Drive Logging Loop" {
    tunnel: w26 -> [w293]
    tunnel: w25 -> [w292]
    tunnel: w13 -> [w291]
    stop <- FALSE stop-if-true
    n149 = local read "Save Drive"() -> (w289:bool)
    n150 = local read "Burst"() -> (w287:i32)
    n151 = call "Drive Data Logger.vi"("Save"=w289, "Array"=w292, "Burst"=w287, "rt fifo"=w293, "TDMS Refnum"=w291) -> ()  [unwired: 7 in]
    n152 = Wait (ms)(milliseconds to wait="loop period (ms) 2") -> ()  [unwired: 1 out]
  }
  n153 = call <vilib>:"WPI_GyroRefNum Registry Get.vi"("refnum name"="yawGyro") -> ("GyroDevRef"=w55:T31)  [unwired: 9 in, 1 out]
  n154 = while {
    tunnel: w55 -> [w294]
    stop <- FALSE stop-if-true
    n155 = case shown="False" "Reset Gyro" {
      tunnel: w294 -> [w298 w300]
      frame True {
        n156 = call <vilib>:"WPI_GyroReset.vi"("GyroDevRef"=w298) -> ()  [unwired: 9 in, 2 out]
      }
      frame False {
        n157 = call <vilib>:"WPI_GyroGetAngle.vi"("GyroDevRef"=w300) -> ("Angle"=w299:dbl)  [unwired: 7 in, 3 out]
        "Angle" <- w299
        n158 = shared-variable ".\\Untitled Library 2.lvlib\\Sensors-Actuators.lvlib\\Gyro.lvlib\\yawGyro"(w299) -> ()  [unwired: 1 in, 1 out]
      }
    }
    n159 = Wait (ms)(milliseconds to wait=u32 40) -> ()  [unwired: 1 out]
  }
  n160 = Bundle(w56, w58, w58, w56, w56) -> (w57:cluster{bool, sgl, sgl, bool, bool})  [unwired: 1 in]
  n161 = local write "Valid Target"(w56) -> ()
  n162 = local write "Valid Ball"(w56) -> ()
  n163 = Type Cast(x=w57) -> (*(type *) &x=w60:string)  [unwired: 1 in]
  n164 = String Length(string=w60) -> (length=w59:i32)
  n165 = UDP Open(11:w65) -> (port=w63:refnum<k16>, 0:w64:errorcluster)  [unwired: 4 in, 1 out]
  n166 = while {
    tunnel: w64 -> [w308]
    tunnel: w63 -> [w307]
    tunnel: [w305] -> w62
    tunnel: [w304] -> w61
    tunnel: w59 -> [w302]
    tunnel: w57 -> [w301]
    stop <- FALSE stop-if-true
    # "Read from com port"
    n167 = UDP Read(connection ID=w307, max size (548)=548, timeout ms (25000)=-1, 8:w308) -> (data out=w303:string, error out=w305:errorcluster, 3:w304:refnum<k16>)  [unwired: 2 out]
    n168 = case shown="No Error" w305 {
      tunnel: w303 -> [w316 _]
      tunnel: w302 -> [w315 _]
      tunnel: w301 -> [w312 _]
      frame No Error {
        # "Cast what is read\n into a cluster"
        # "Ensure what is read matches the type"
        n169 = Type Cast(type=w312, x=w316) -> (*(type *) &x=w311:cluster{bool, sgl, sgl, bool, bool})
        n170 = String Length(string=w316) -> (length=w314:i32)
        n171 = Equal?(x=w314, y=w315) -> (x = y?=w313:bool)
        n172 = case shown="True" w313 {
          tunnel: w311 -> [_ w322]
          frame False {
          }
          frame True {
            n173 = Unbundle(w322) -> (w319:bool, w318:sgl, w317:sgl, w320:bool, w321:bool)
            "Valid Ball" <- w319
            "Ball X" <- w318
            "Ball Y" <- w317
            "Valid Target" <- w320
            "Direction" <- w321
            n174 = shared-variable ".\\Untitled Library 2.lvlib\\Vision.lvlib\\Valid Target"(w320) -> ()  [unwired: 1 in, 1 out]
            n175 = shared-variable ".\\Untitled Library 2.lvlib\\Vision.lvlib\\Direction"(w321) -> ()  [unwired: 1 in, 1 out]
            n176 = shared-variable ".\\Untitled Library 2.lvlib\\Vision.lvlib\\Ball Y"(w317) -> ()  [unwired: 1 in, 1 out]
            n177 = shared-variable ".\\Untitled Library 2.lvlib\\Vision.lvlib\\Valid Ball"(w319) -> ()  [unwired: 1 in, 1 out]
            n178 = shared-variable ".\\Untitled Library 2.lvlib\\Vision.lvlib\\Ball X"(w318) -> ()  [unwired: 1 in, 1 out]
          }
        }
      }
      frame Error {
      }
    }
  }
  n179 = disable-structure shown="Disabled" {
    frame Disabled {
      # "Auto-turn"
      n180 = while {
        stop <- FALSE stop-if-true
        n181 = feedback #1() -> (w327:dbl)  [unwired: 1 in]
        n182 = feedback #2(enum16{"Wait", "Turn Left", "Turn Right"}."Wait") -> (w329:enum16{"Wait", "Turn Left", "Turn Right"})
        n183 = case shown="\"Turn Left\"" w329 {
          tunnel: [w340 w347 w356] -> w328
          tunnel: w327 -> [_ w347 w356]
          tunnel: [w333 w348 w357] -> w326
          tunnel: "Turn" -> [_ w345 w358]
          tunnel: "Turn Time" -> [_ w346 w355]
          frame "Wait", Default {
            n184 = Get Date/Time In Seconds() -> (seconds since 1Jan1904=w341:timestamp)
            n185 = shared-variable ".\\Untitled Library 2.lvlib\\Operator.lvlib\\operatorButton5"() -> (w339:bool)  [unwired: 1 in, 1 out]
            n186 = shared-variable ".\\Untitled Library 2.lvlib\\Driver.lvlib\\driverJoystickAxis3"(0.0 ("driverJoystickAxis3")) -> ()  [unwired: 1 in, 1 out]
            n187 = To Double Precision Float(number=w341) -> (double precision float=w340:dbl)
            n188 = shared-variable ".\\Untitled Library 2.lvlib\\Operator.lvlib\\operatorButton6"() -> (w335:bool)  [unwired: 1 in, 1 out]
            n189 = Select(t=enum16{"Wait", "Turn Left", "Turn Right"}."Turn Left", s=w339, f=enum16{"Wait", "Turn Left", "Turn Right"}."Wait") -> (s? t:f=w336:enum16{"Wait", "Turn Left", "Turn Right"})
            n190 = Select(t=enum16{"Wait", "Turn Left", "Turn Right"}."Turn Right", s=w335, f=w336) -> (s? t:f=w333:enum16{"Wait", "Turn Left", "Turn Right"})
          }
          frame "Turn Left" {
            n191 = Get Date/Time In Seconds() -> (seconds since 1Jan1904=w353:timestamp)
            n192 = Negate(x=w345) -> (-x=w343:dbl)
            n193 = Add(x=w347, y=w346) -> (x+y=w354:dbl)
            n194 = To Double Precision Float(number=w353) -> (double precision float=w352:dbl)
            n195 = Add(x=w343, y="Left Turn Offset") -> (x+y=w344:dbl)
            n196 = Greater?(x=w354, y=w352) -> (0:w351:bool)
            n197 = shared-variable ".\\Untitled Library 2.lvlib\\Driver.lvlib\\driverJoystickAxis3"(w344) -> ()  [unwired: 1 in, 1 out]
            n198 = Select(t=enum16{"Wait", "Turn Left", "Turn Right"}."Turn Left", s=w351, f=enum16{"Wait", "Turn Left", "Turn Right"}."Wait") -> (s? t:f=w348:enum16{"Wait", "Turn Left", "Turn Right"})
          }
          frame "Turn Right" {
            n199 = Get Date/Time In Seconds() -> (seconds since 1Jan1904=w363:timestamp)
            n200 = Add(x=w356, y=w355) -> (x+y=w364:dbl)
            n201 = To Double Precision Float(number=w363) -> (double precision float=w362:dbl)
            n202 = Greater?(x=w364, y=w362) -> (0:w361:bool)
            n203 = shared-variable ".\\Untitled Library 2.lvlib\\Driver.lvlib\\driverJoystickAxis3"(w358) -> ()  [unwired: 1 in, 1 out]
            n204 = Select(t=enum16{"Wait", "Turn Left", "Turn Right"}."Turn Right", s=w361, f=enum16{"Wait", "Turn Left", "Turn Right"}."Wait") -> (s? t:f=w357:enum16{"Wait", "Turn Left", "Turn Right"})
          }
        }
        n205 = feedback-in #1(w328) -> ()
        n206 = feedback-in #2(w326) -> ()
        n207 = Wait (ms)(milliseconds to wait=u32 30) -> ()  [unwired: 1 out]
      }
    }
    frame Enabled {
    }
  }
  n208 = UDP Close(connection ID=w61, 8:w62) -> ()  [unwired: 2 out]
  n209 = Get Date/Time In Seconds() -> (seconds since 1Jan1904=w29:timestamp)
  n210 = To Double Precision Float(number=w29) -> (double precision float=w28:dbl)
  n211 = while {
    tunnel: w40 -> [w397]
    tunnel: w37 -> [w408]
    tunnel: w36 -> [w407]
    tunnel: w25 -> [w392]
    tunnel: w28 -> [w391]
    tunnel: w26 -> [w390]
    stop <- FALSE stop-if-true
    n212 = shared-variable ".\\Untitled Library 2.lvlib\\Misc..lvlib\\autoTurn?"() -> (w371:bool)  [unwired: 1 in, 1 out]
    n213 = call "Dual Sonar and Perpendicular Distance.vi"("Sonar Offset"="Sonar Offset 2", "Left Sonar Dev Ref"=w408, "Sonar Scale"="Sonar Scale 2", "Radius of Ball"=12.5, "Right Sonar Dev Ref"=w407, "ResetSonar"="Reset Sonar 2") -> ("Left"=→"Left 2":dbl, "Right"=→"Right 2":dbl, "Perpendicular Distance to Ball"=→"Perpendicular Distance to Ball 2":dbl)
    n214 = shared-variable ".\\Untitled Library 2.lvlib\\Driver.lvlib\\driverButton9"() -> (w396:bool)  [unwired: 1 in, 1 out]
    n215 = shared-variable ".\\Untitled Library 2.lvlib\\Driver.lvlib\\driverButton3"() -> (w389:bool)  [unwired: 1 in, 1 out]
    n216 = shared-variable ".\\Untitled Library 2.lvlib\\Sensors-Actuators.lvlib\\Gyro.lvlib\\Desired Angle"() -> (w372:dbl)  [unwired: 1 in, 1 out]
    n217 = shared-variable ".\\Untitled Library 2.lvlib\\Driver.lvlib\\driverButton4"() -> (w381:bool)  [unwired: 1 in, 1 out]
    n218 = Select(t=T32."Rotate" ("Drive Mode"), s=w371, f=T32."Distance Drive" ("Drive Mode")) -> (s? t:f=w375:T32)
    n219 = Select(t=w375, s=w396, f=T32."Drive" ("Drive Mode")) -> (s? t:f=w395:T32)
    n220 = shared-variable ".\\Untitled Library 2.lvlib\\Sensors-Actuators.lvlib\\Motor.lvlib\\EncoderRightDistance"() -> (w370:dbl)  [unwired: 1 in, 1 out]
    n221 = shared-variable ".\\Untitled Library 2.lvlib\\Driver.lvlib\\driverJoystickAxis1"() -> (w384:dbl)  [unwired: 1 in, 1 out]
    n222 = shared-variable ".\\Untitled Library 2.lvlib\\Driver.lvlib\\driverJoystickAxis2"() -> (w383:dbl)  [unwired: 1 in, 1 out]
    n223 = shared-variable ".\\Untitled Library 2.lvlib\\Driver.lvlib\\driverJoystickAxis3"() -> (w382:dbl)  [unwired: 1 in, 1 out]
    n224 = shared-variable ".\\Untitled Library 2.lvlib\\Sensors-Actuators.lvlib\\Motor.lvlib\\Encoder LeftDistance"() -> (w369:dbl)  [unwired: 1 in, 1 out]
    n225 = Select(t=T32."Track X" ("Drive Mode"), s=w389, f=w395) -> (s? t:f=w378:T32)
    n226 = shared-variable ".\\Untitled Library 2.lvlib\\Sensors-Actuators.lvlib\\Gyro.lvlib\\yawGyro"() -> (w380:dbl)  [unwired: 1 in, 1 out]
    "yawGyro" <- w380
    "yawGyro 2" <- w380
    n227 = shared-variable ".\\Untitled Library 2.lvlib\\Misc..lvlib\\desiredDriveDistance"() -> (w368:dbl)  [unwired: 1 in, 1 out]
    n228 = shared-variable ".\\Untitled Library 2.lvlib\\Vision.lvlib\\Valid Ball"() -> (w367:bool)  [unwired: 1 in, 1 out]
    n229 = shared-variable ".\\Untitled Library 2.lvlib\\Vision.lvlib\\Ball X"() -> (w366:dbl)  [unwired: 1 in, 1 out]
    n230 = call "Drive-Rotate-Camera_Track.vi"("Ball X"=w366, "Valid Ball?"=w367, "Desisred Distance"=w368, "Left Encoder"=w369, "Right Encoder"=w370, "Drive Mode"=w378, "Controller X"=w384, "Controller Y"=w383, "Controller Rotate"=w382, "Strafe?"=w381, "Eval Period (sec)"="Eval Period (sec)", "Gyro Angle"=w380, "Desired Angle"=w372) -> ("Rotate Out"=w386:dbl, "X Out"=w385:dbl, "Y Out"=w387:dbl, "Stable"=w365:bool)  [unwired: 3 in]
    "Stable" <- w365
    n231 = case shown="True" "Tank Test" {
      tunnel: w397 -> [w432 w442]
      tunnel: w380 -> [_ w441]
      tunnel: w387 -> [w431 _]
      tunnel: w386 -> [w430 _]
      tunnel: w385 -> [w429 _]
      frame False {
        n232 = call-poly <vilib>:"WPI_RobotDriveHolonomicDrive.vi"("Rotation"=w430, "Y"=w431, "X"=w429, "RobotDriveDevRef"=w432) -> ()  [unwired: 5 in, 3 out]
      }
      frame True {
        n233 = Negate(x="Limit") -> (-x=w436:dbl)
        n234 = Bundle("Limit"="Limit", w436) -> (w434:cluster{"Limit":dbl, dbl})  [unwired: 1 in]
        n235 = call-poly <vilib>:"PID.vi"("output range"=w434, "PID gains"="PID gains", "process variable"=w441) -> ("output"=w438:dbl)  [unwired: 7 in, 1 out]
        n236 = call "Differential Steering.vi"("Steer"=w438, "Base"="Base") -> ("Right"=w439:dbl, "Left"=w440:dbl)  [unwired: 4 in]
        n237 = call <vilib>:"WPI_RobotDriveTankDrive.vi"("Right axis value"=w439, "Left axis value"=w440, "RobotDriveDevRef"=w442) -> ()  [unwired: 6 in, 3 out]
      }
    }
    n238 = shared-variable ".\\Untitled Library 2.lvlib\\Misc..lvlib\\Drive Stable?"(w365) -> ()  [unwired: 1 in, 1 out]
    n239 = Subtract(x=w372, y=w380) -> (x-y=→"Auto Turn Error":dbl)
    n240 = Wait (ms)(milliseconds to wait=u32 20) -> ()  [unwired: 1 out]
    n241 = case shown="True" "Log Enable" {
      tunnel: w392 -> [_ w418]
      tunnel: w391 -> [_ w417]
      tunnel: w390 -> [_ w416]
      tunnel: w380 -> [_ w415]
      tunnel: w389 -> [_ w414]
      frame False {
      }
      frame True {
        (unwired) 1 ("index")
        (unwired) 0 ("index")
        n242 = Get Date/Time In Seconds() -> (seconds since 1Jan1904=w427:timestamp)
        n243 = Boolean To (0,1)(Boolean=w414) -> (0, 1=w413:i16)
        n244 = To Double Precision Float(number=w427) -> (double precision float=w428:dbl)
        n245 = Subtract(x=w428, y=w417) -> (x-y=w409:dbl)
        n246 = feedback #3(u32 0 ("# elements")) -> (w425:u32)
        n247 = Replace Array Subset(array=w418, new element #1=w409, index #1=0 ("index"), new element #2=w415, index #2=1 ("index"), new element #3=w413, index #3=2 ("index"), new element #4=w413, index #4=3 ("index"), new element #5=w425, index #5=4 ("index")) -> (w423:dbl[])
        n248 = RT FIFO Write(0:w416, 1:w423) -> (7:w412:u32)  [unwired: 3 in, 3 out]
        n249 = feedback-in #3(w412) -> ()
        n250 = Greater?(x=w412, y="Burst") -> (0:→"Save Drive":bool)
      }
    }
  }
